vi "pdv_usb1.vi"() -> ()   [LabVIEW 2010]
uses:
  70user.lib/TheSigTab.vi
  <vilib>/Utility/config.llb/Read Key (U32).vi
  <vilib>/Utility/config.llb/Read Key (Boolean).vi
  <vilib>/Utility/config.llb/Read Key (Double).vi
  <vilib>/addons/database/Connection.llb/DB Tools Open Connec (Path).vi
  <vilib>/Utility/config.llb/Read Key (String).vi
  <vilib>/Utility/config.llb/Write Key (Double).vi
  <vilib>/Utility/config.llb/Write Key (U32).vi
  <vilib>/Utility/config.llb/Write Key (Boolean).vi
  <vilib>/addons/database/NI_Database_API.lvlib
  <vilib>/Utility/config.llb/NI_LVConfig.lvlib
panel:
  in  "ScopeToo":bool caption="Сохранять осциллограммы"
  in  "m_s":u16(ring) items=["мин", "сек"]
  in  "Object":string(combo) caption="Объект"
  in  "CurvesToo":bool caption="Сохранять графики"
  in  "AcqureTime":dbl caption="опроса" format="%#.3g"
  out "ExtDev":bool caption="Выносной модуль"
  in  "SaveTime":dbl=1.0 caption="мин" min=1.0 max=120.0
  out "Slide":u8(slide) scale=0.0..100.0
  in  "Continuosly":bool caption="Периодически"
  in  "SaveNow":bool caption="Однократно"
  in  "Loop":bool caption="Зациклить данные"
  out "Current time":timestamp caption="Время и Дата" format="%<%X\n%x>T"
  out "Tper":dbl caption="общая"
  in  "filter":bool caption="Фильтр\nперекрёстных помех"
  in  "Stop":bool
  in  "Table":string[][](table) caption="Результаты измерений"
  # "Запись в базу данных"
  # "Продолжительность, с"
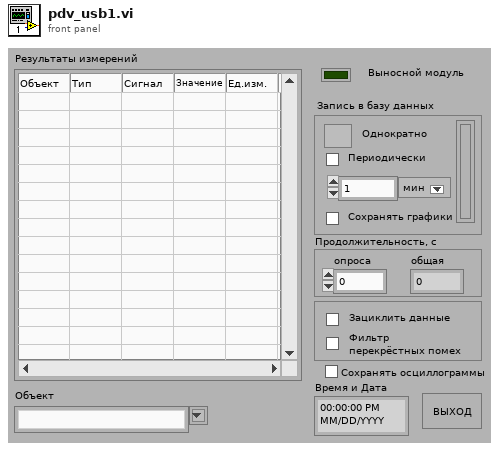
[diagram p1: front panel]
types:
  T1 = typedef "NI_LVConfig.lvlib/Config Data RefNum.ctl" = refnum<k1>
  T2 = typedef "NI_Database_API.lvlib/Conn ObjectReference.ctl" = refnum<k1>
  T3 = cluster{"Status":bool, "ViErrorNumber":u32, "ViName":string, "ViErrorString":string, "CinName":string, "CinErrorString":string}
  T4 = cluster{"VirtualSlot":u16, "ModuleName":string, "SerialNumber":string, "UsbSpeed":u8, "AvrVersion":string, "ModuleRevision":string, "DspType":string, "IsDacPresented":bool, "DspLoading":bool, "DspVersion":string, "DspClockout":u32, "AdcOffsetCoef":sgl[], "AdcScaleCoef":sgl[], "DacOffsetCoef":sgl[], "DacScaleCoef":sgl[]}
  T5 = cluster{"DllVersion":u32, "InterfaceType":u32, "InterfaceInstance":u32, "ModuleHandle":u32, "ReadBuffersParsArray":cluster{"Buffer":i16[], "ReadOv":u32, "ReadEvent":u32}[], "WriteBuffersParsArray":cluster{"Buffer":i16[], "WriteOv":u32, "WriteEvent":u32}[]}
  T6 = cluster{"Сигнал":string, "Тип":enum16{"Напряжение/Ток", "ЧР", "Температура", "Давление"}, "Object":string}[]
  T7 = cluster{"Сигнал":string, "Тип":enum16{"Напряжение/Ток", "ЧР", "Температура", "Давление"}, "Object":string}
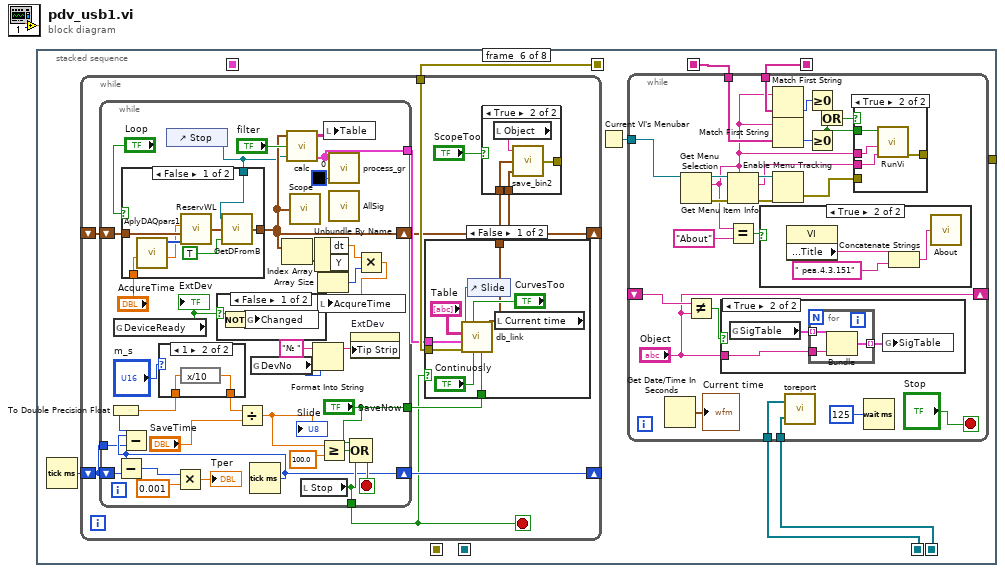
[diagram p0: block diagram]
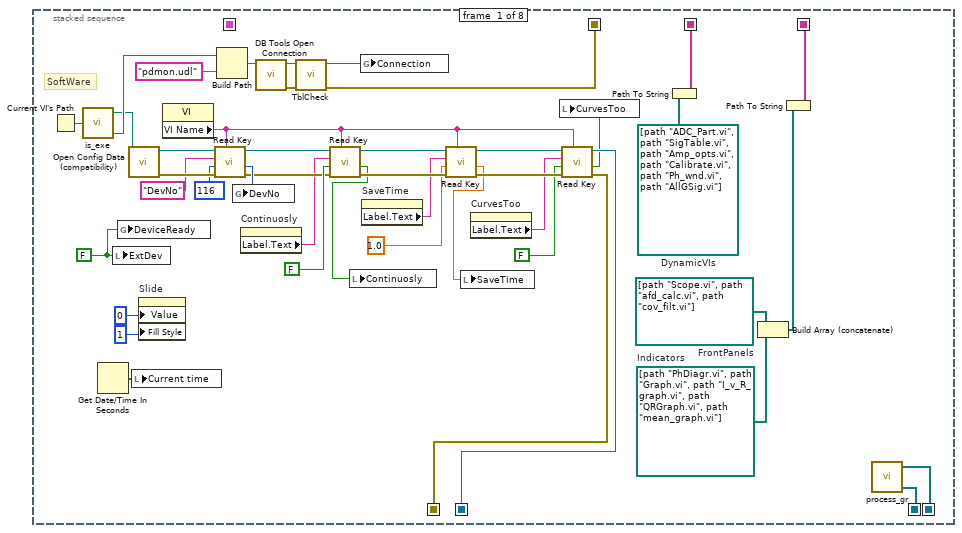
[diagram p2: hidden frame]
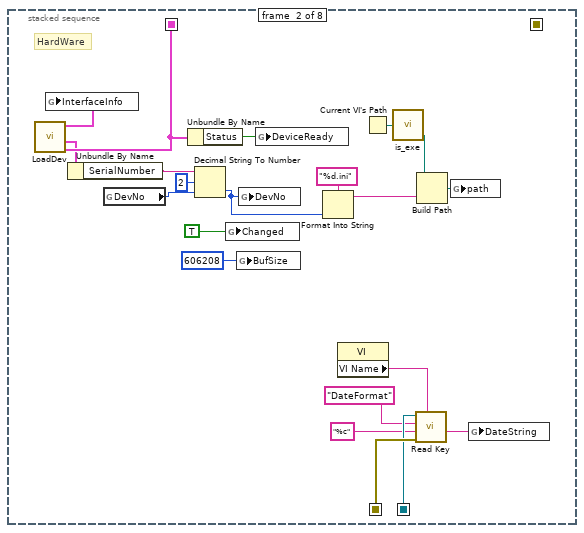
[diagram p3: hidden frame]
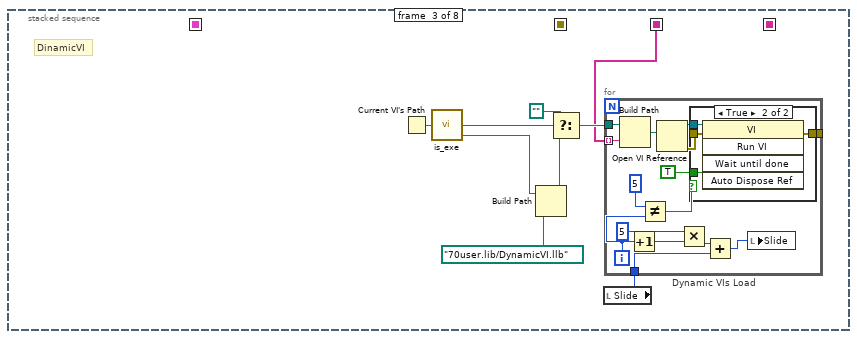
[diagram p4: hidden frame]
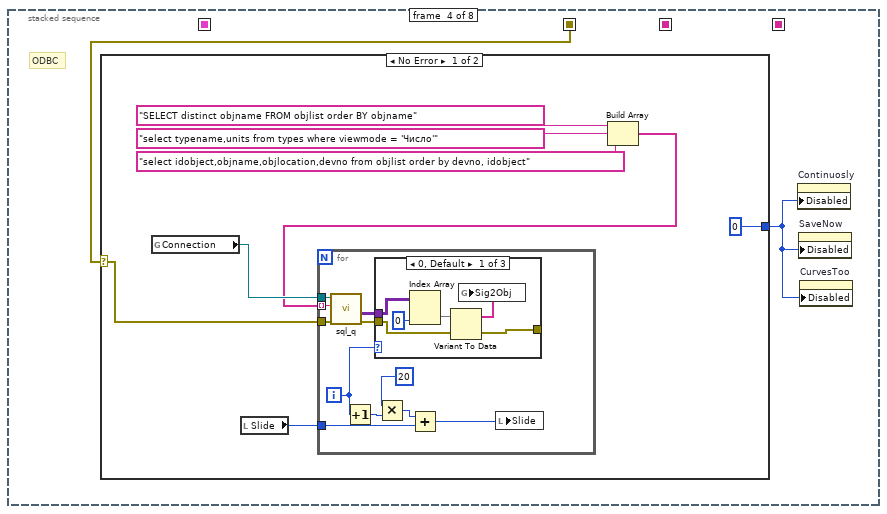
[diagram p6: hidden frame]
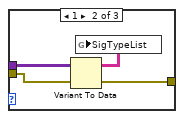
[diagram p7: hidden frame]
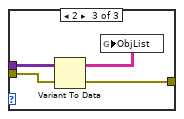
[diagram p8: hidden frame]
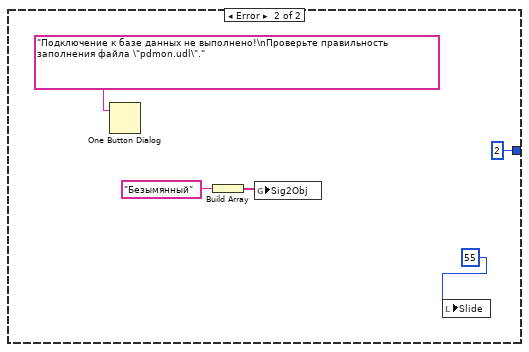
[diagram p9: hidden frame]
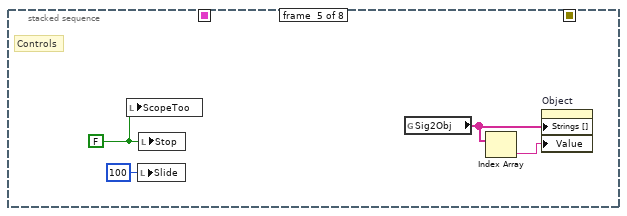
[diagram p10: hidden frame]
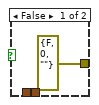
[diagram p11: hidden frame]
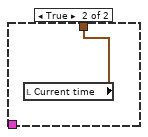
[diagram p12: hidden frame]
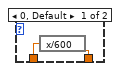
[diagram p13: hidden frame]
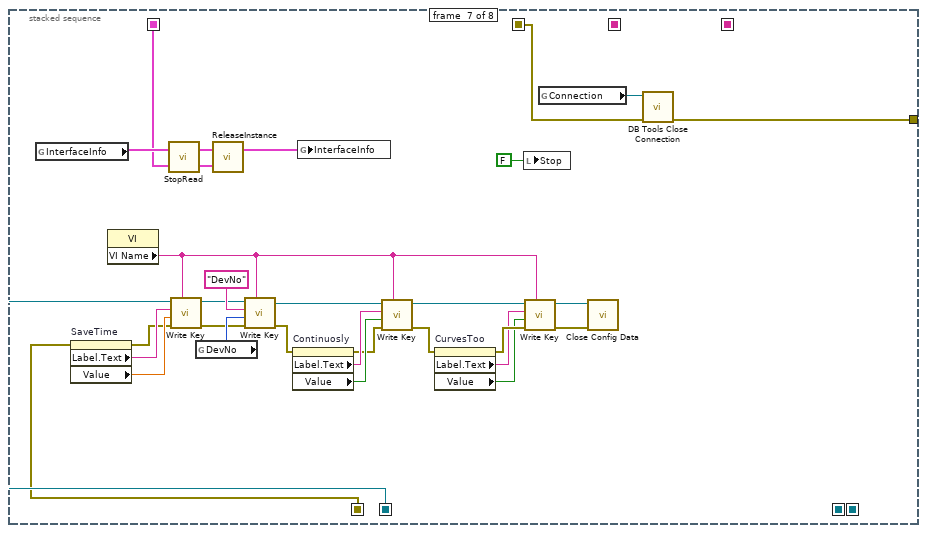
[diagram p19: hidden frame]
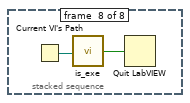
[diagram p20: hidden frame]
diagram:
  n1 = stacked-sequence {
    seq-local: [_ w60 _ _ _ _ _ _] -> [_ _ _ _ _ _ w282 _]
    seq-local: [w30 _ _ _ _ _ _ _] -> [_ _ _ w96 _ w144 w289 _]
    seq-local: [w33 _ _ _ _ _ _ _] -> [_ _ _ _ _ w142 _ _]
    seq-local: [w37 _ _ _ _ _ _ _] -> [_ _ w69 _ _ w141 _ _]
    seq-local: [w40 _ _ _ _ _ _ _] -> [_ _ _ _ _ w139 _ _]
    seq-local: [w39 _ _ _ _ _ _ _] -> [_ _ _ _ _ w140 _ _]
    seq-local: [w9 _ _ _ _ _ _ _] -> [_ w49 _ _ _ _ w274 _]
    seq-local: [w10 _ _ _ _ _ _ _] -> [_ w50 _ _ _ _ w268 _]
    tunnel: [_ _ _ _ _ _ w286 _] -> _
    frame #0 {
      w19 = FALSE ("ExtDev")
      w35 = path[] [path "PhDiagr.vi", path "Graph.vi", path "I_v_R_graph.vi", path "QRGraph.vi", path "mean_graph.vi"]  # Indicators
      w36 = path[] [path "Scope.vi", path "afd_calc.vi", path "cov_filt.vi"]  # FrontPanels
      w38 = path[] [path "ADC_Part.vi", path "SigTable.vi", path "Amp_opts.vi", path "Calibrate.vi", path "Ph_wnd.vi", path "AllGSig.vi"]  # DynamicVIs
      # "SoftWare"
      n2 = Current VI's Path() -> (path=w44:path)
      n3 = call "is_exe.vi"("path"=w44) -> ("actual path"=w43:path, "ini path"=w25:path)  [unwired: 2 in, 1 out]
      n4 = Get Date/Time In Seconds() -> (seconds since 1Jan1904=w28:timestamp)
      n5 = local write "ExtDev"(w19) -> ()
      n6 = global write "TheSigTab.vi" "DeviceReady"(w19) -> ()
      n7 = call <vilib>:"Open Config Data (compatibility).vi"("configuration file path"=w25) -> ("error out"=w23:errorcluster, "refnum"=w24:T1)  [unwired: 8 in, 1 out]
      n8 = local write "Current time"(w28) -> ()
      n9 = property on="Slide" class="Slide (strict)"("Value"=u8 0 ("Slide"), "Fill Style"=1) -> ()  [unwired: 2 in, 2 out]
      n10 = property class="VI"() -> ("VI Name"=w17:string)  [unwired: 2 in, 2 out]
      n11 = call-poly <vilib>:"Read Key.vi"("section"=w17, "error in (no error)"=w23, "default value"=u32 116 ("DevNo"), "key"="DevNo", "refnum"=w24) -> ("error out"=w15:errorcluster, "value"=w20:u32, "refnum out"=w18:T1)  [unwired: 3 in, 1 out]
      n12 = Build Path(base path=w43, name or relative path="pdmon.udl") -> (appended path=w41:path)
      n13 = global write "TheSigTab.vi" "DevNo"(w20) -> ()
      n14 = property on="Continuosly" class="Bool (strict)"() -> ("Label.Text"=w4:string)  [unwired: 2 in, 2 out]
      n15 = call-poly <vilib>:"DB Tools Open Connection.vi"("connection information"=w41) -> ("error out"=w31:errorcluster, "connection reference"=w32:T2)  [unwired: 7 in]
      n16 = call "TblCheck.vi"("error in"=w31, "connection reference"=w32) -> ("error out"=w30:errorcluster, "conn ref out"=w29:T2)  [unwired: 3 in, 1 out]
      n17 = call-poly <vilib>:"Read Key.vi"("section"=w17, "error in (no error)"=w15, "default value"=FALSE, "key"=w4, "refnum"=w18) -> ("error out"=w14:errorcluster, "value"=w2:bool, "refnum out"=w12:T1)  [unwired: 3 in, 1 out]
      n18 = local write "Continuosly"(w2) -> ()
      n19 = global write "TheSigTab.vi" "Connection"(w29) -> ()
      n20 = property on="SaveTime" class="DigNum (strict)"() -> ("Label.Text"=w3:string)  [unwired: 2 in, 2 out]
      n21 = call-poly <vilib>:"Read Key.vi"("section"=w17, "error in (no error)"=w14, "default value"=1.0, "key"=w3, "refnum"=w12) -> ("error out"=w13:errorcluster, "value"=w6:dbl, "refnum out"=w11:T1)  [unwired: 3 in, 1 out]
      n22 = local write "SaveTime"(w6) -> ()
      n23 = property on="CurvesToo" class="Bool (strict)"() -> ("Label.Text"=w1:string)  [unwired: 2 in, 2 out]
      n24 = call-poly <vilib>:"Read Key.vi"("section"=w17, "error in (no error)"=w13, "default value"=FALSE, "key"=w1, "refnum"=w11) -> ("error out"=w10:errorcluster, "value"=w5:bool, "refnum out"=w9:T1)  [unwired: 3 in, 1 out]
      n25 = local write "CurvesToo"(w5) -> ()
      n26 = Path To String(path=w38) -> (string=w37:string[])
      n27 = Build Array (concatenate)(w36, w35) -> (w34:path[])
      n28 = Path To String(path=w34) -> (string=w33:string[])
      n29 = call "process_gr.vi"() -> ("WG refs"=w40:refnum<vi>[], "menu refs"=w39:refnum<k9>[])  [unwired: 4 in]
    }
    frame #1 {
      # "HardWare"
      n30 = call "LoadDev.vi"() -> ("ViStatus"=w60:T3, "ModuleInfo"=w59:T4, "InterfaceInfo"=w61:T5)  [unwired: 5 in]
      n31 = global write "TheSigTab.vi" "InterfaceInfo"(w61) -> ()
      n32 = Unbundle By Name(w59) -> ("SerialNumber"=w58:string)
      n33 = global read "TheSigTab.vi" "DevNo"() -> (w51:u32)
      n34 = Unbundle By Name(w60) -> ("Status"=w65:bool)
      n35 = Decimal String To Number(string=w58, offset=u32 2 ("initial scan location"), default (0L)=w51) -> (number=w53:u32)  [unwired: 1 out]
      n36 = global write "TheSigTab.vi" "Changed"(TRUE ("Changed")) -> ()
      n37 = global write "TheSigTab.vi" "BufSize"(u32 606208 ("BufSize")) -> ()
      n38 = global write "TheSigTab.vi" "DevNo"(w53) -> ()
      n39 = global write "TheSigTab.vi" "DeviceReady"(w65) -> ()
      n40 = Format Into String(format string="%d.ini", w53) -> (resulting string=w55:string)  [unwired: 2 in, 1 out]
      n41 = property class="VI"() -> ("VI Name"=w48:string)  [unwired: 2 in, 2 out]
      n42 = Current VI's Path() -> (path=w64:path)
      n43 = call "is_exe.vi"("path"=w64) -> ("actual path"=w52:path)  [unwired: 2 in, 2 out]
      n44 = call-poly <vilib>:"Read Key.vi"("section"=w48, "error in (no error)"=w50, "default value"="%c", "key"="DateFormat", "refnum"=w49) -> ("value"=w45:string)  [unwired: 3 in, 3 out]
      n45 = Build Path(base path=w52, name or relative path=w55) -> (appended path=w54:path)
      n46 = global write "TheSigTab.vi" "path"(w54) -> ()
      n47 = global write "TheSigTab.vi" "DateString"(w45) -> ()
    }
    frame #2 {
      # "DinamicVI"
      n48 = Current VI's Path() -> (path=w68:path)
      n49 = call "is_exe.vi"("path"=w68) -> ("actual path"=w66:path, "exe?"=w67:bool)  [unwired: 2 in, 1 out]
      n50 = Build Path(base path=w66, name or relative path=path "70user.lib/DynamicVI.llb" ("f")) -> (appended path=w70:path)
      n51 = Select(t=path "", s=w67, f=w70) -> (s? t:f=w74:path)
      n52 = local read "Slide"() -> (w73:u8)
      n53 = for "Dynamic VIs Load" {
        tunnel: w69 -> [w89] mode=indexing
        tunnel: w74 -> [w87]
        tunnel: w73 -> [w83]
        tunnel: [w78] -> _
        i -> [w77]
        n54 = Build Path(base path=w87, name or relative path=w89) -> (appended path=w88:path)
        n55 = Increment(x=w77) -> (x+1=w79:i32)
        n56 = Not Equal?(x=5, y=w77) -> (x != y?=w75:bool)
        n57 = Open VI Reference(vi path=w88) -> (vi reference=w85:refnum<vi>, error out=w84:errorcluster)  [unwired: 5 in]
        n58 = Multiply(x=5, y=w79) -> (x*y=w81:i32)
        n59 = case shown="True" w75 {
          tunnel: TRUE ("Wait until done") -> [_ w94]
          tunnel: w85 -> [_ w93]
          tunnel: w84 -> [w90 w92]
          tunnel: [w90 w91] -> w78
          frame False {
          }
          frame True {
            n60 = invoke class="VI" method="Run VI"(reference=w93, error in=w92, "Wait until done"=w94) -> (error out=w91:errorcluster)  [unwired: 2 in, 4 out]
          }
        }
        n61 = Add(x=w81, y=w83) -> (x+y=w82:i32)
        n62 = local write "Slide"(w82) -> ()
      }
    }
    frame #3 {
      # "ODBC"
      n63 = case shown="No Error" w96 {
        selector: w96 -> [w100 _]
        tunnel: [u8 0 ("Disabled") u8 2 ("Disabled")] -> w95
        frame No Error {
          n64 = global read "TheSigTab.vi" "Connection"() -> (w101:T2)
          n65 = local read "Slide"() -> (w98:u8)
          n66 = Build Array("SELECT distinct objname FROM objlist order BY objname", "select typename,units from types where viewmode = 'Число'", "select idobject,objname,objlocation,devno from objlist order by devno, idobject" ("table")) -> (w99:string[])
          n67 = for {
            tunnel: w101 -> [w114]
            tunnel: w100 -> [w113]
            tunnel: w99 -> [w111] mode=indexing
            tunnel: w98 -> [w110]
            i -> [w107]
            n68 = call "sql_q.vi"("error in"=w113, "SQL query"=w111, "connect ref"=w114) -> ("error out"=w112:errorcluster, "recordset data"=w115:variant[][])  [unwired: 1 in, 2 out]
            n69 = Increment(x=w107) -> (x+1=w105:i32)
            n70 = case shown="0, Default" w107 {
              tunnel: w115 -> [w118 w125 w129]
              tunnel: w112 -> [w117 w123 w127]
              tunnel: [w116 w122 w126] -> _
              frame 0, Default {
                n71 = Index Array(array=w118, index (col)=0 ("disabled index (col)")) -> (element=w120:variant[])  [unwired: 1 in]
                n72 = Variant To Data(error in=w117, Variant=w120) -> (error out=w116:errorcluster, data=w119:string[])  [unwired: 1 in]
                n73 = global write "TheSigTab.vi" "Sig2Obj"(w119) -> ()
              }
              frame 1 {
                n74 = Variant To Data(error in=w123, Variant=w125) -> (error out=w122:errorcluster, data=w124:string[][])  [unwired: 1 in]
                n75 = global write "TheSigTab.vi" "SigTypeList"(w124) -> ()
              }
              frame 2 {
                n76 = Variant To Data(error in=w127, Variant=w129) -> (error out=w126:errorcluster, data=w128:string[][])  [unwired: 1 in]
                n77 = global write "TheSigTab.vi" "ObjList"(w128) -> ()
              }
            }
            n78 = Multiply(x=20, y=w105) -> (x*y=w108:i32)
            n79 = Add(x=w108, y=w110) -> (x+y=w109:i32)
            n80 = local write "Slide"(w109) -> ()
          }
        }
        frame Error {
          n81 = One Button Dialog(message="Подключение к базе данных не выполнено!\nПроверьте правильность заполнения файла \"pdmon.udl\".") -> ()  [unwired: 1 in, 1 out]
          n82 = Build Array("Безымянный" ("table")) -> (w133:string[])
          n83 = global write "TheSigTab.vi" "Sig2Obj"(w133) -> ()
          n84 = local write "Slide"(u8 55 ("Slide")) -> ()
        }
      }
      n85 = property on="Continuosly" class="Bool (strict)"("Disabled"=w95) -> ()  [unwired: 2 in, 2 out]
      n86 = property on="SaveNow" class="Bool"("Disabled"=w95) -> ()  [unwired: 2 in, 2 out]
      n87 = property on="CurvesToo" class="Bool (strict)"("Disabled"=w95) -> ()  [unwired: 2 in, 2 out]
    }
    frame #4 {
      w135 = FALSE ("Changed")
      # "Controls"
      n88 = local write "ScopeToo"(w135) -> ()
      n89 = local write "Slide"(u8 100 ("Slide")) -> ()
      n90 = local write "Stop"(w135) -> ()
      n91 = global read "TheSigTab.vi" "Sig2Obj"() -> (w137:string[])
      n92 = Index Array(array=w137) -> (element=w136:string)  [unwired: 1 in]
      n93 = property on="Object" class="CmbBox"("Strings []"=w137, "Value"=w136) -> ()  [unwired: 2 in, 2 out]
    }
    frame #5 {
      n94 = Tick Count (ms)() -> (millisecond timer value=w145:u32)
      n95 = while {
        shift-right: [w155] -> _
        shift-left: w145 -> [w152]
        shift-right: [w148] -> _
        shift-left: _ -> [w154]
        tunnel: w144 -> [w153]
        stop <- w149 stop-if-true
        n96 = while {
          shift-right: [w182] -> w148
          shift-left: w154 -> [w201]
          shift-right: [w196] -> w155
          shift-left: w152 -> [w202]
          tunnel: [w198] -> w149
          tunnel: w152 -> [w195]
          tunnel: ["SaveNow"] -> w151
          tunnel: [w188] -> w150
          stop <- w197 stop-if-true
          n97 = global read "TheSigTab.vi" "DeviceReady"() -> (w193:bool)
          "ExtDev" <- w193
          n98 = control-ref of="Stop"() -> (w176:refnum<vi>)
          n99 = case shown="False" "Loop" {
            tunnel: w201 -> [w218 w219]
            tunnel: [w215 w219] -> w182
            tunnel: "AcqureTime" -> [w212 _]
            tunnel: w176 -> [w211 _]
            frame False {
              n100 = call "AplyDAQpars1.vi"("AcqTimeIn"=w212) -> ("t1-t0"=w213:dbl, "Idxs"=w217:i32[])  [unwired: 5 in]
              n101 = call "ReservWL.vi"("Tags"=w217, "ArrayIn"=w218, "t1-t0"=w213) -> ("Array"=w216:waveform(i16)[])  [unwired: 1 in]
              n102 = call "GetDFromB.vi"("Control"=TRUE, "ArrayIn"=w216, "Bool Refnum"=w211) -> ("ArrayOut"=w215:waveform(i16)[])
            }
            frame True {
            }
          }
          n103 = case shown="False" w193 {
            selector: w193 -> [w210 _]
            frame False {
              n104 = Not(x=w210) -> (.not. x?=w209:bool)
              n105 = global write "TheSigTab.vi" "Changed"(w209) -> ()
            }
            frame True {
            }
          }
          n106 = Tick Count (ms)() -> (millisecond timer value=w196:u32)
          n107 = Subtract(x=w196, y=w202) -> (x-y=w192:u32)
          n108 = Subtract(x=w196, y=w195) -> (x-y=w194:u32)
          n109 = To Double Precision Float(number=w194) -> (double precision float=w171:dbl)
          n110 = case shown="1" "m_s" {
            tunnel: w171 -> [w206 w208]
            tunnel: [w205 w207] -> w170
            frame 0, Default {
              n111 = expression code="x/600"(w206) -> (w205:dbl)
            }
            frame 1 {
              n112 = expression code="x/10"(w208) -> (w207:dbl)
            }
          }
          n113 = Multiply(x=w192, y=0.001 ("x")) -> (x*y=→"Tper":dbl)
          n114 = Divide(x=w170, y="SaveTime") -> (x/y=w186:dbl)
          "Slide" <- w186
          n115 = global read "TheSigTab.vi" "DevNo"() -> (w173:u32)
          n116 = Index Array(array=w182) -> (element=w181:waveform(i16))  [unwired: 1 in]
          n117 = call "calc.vi"("Acquire"=w176, "filter"="filter", "ArrayIn"=w182) -> ("AllMeasures"=w188:cluster{"x0":dbl, "dx":dbl, "y":sgl[][]}[], "Values"=w204:string[][])  [unwired: 1 in]
          n118 = call "Scope.vi"("Array"=w182) -> ()
          n119 = local read "Stop"() -> (w198:bool)
          n120 = Format Into String(initial string="№ ", w173) -> (resulting string=w175:string)  [unwired: 2 in, 1 out]
          n121 = Unbundle By Name(w181) -> ("dt"=w179:dbl, "Y"=w180:i16[])
          n122 = Array Size(array=w180) -> (size(s)=w178:i32)
          n123 = Greater Or Equal?(x=w186, y=100.0 ("x")) -> (x >= y?=w183:bool)
          n124 = local write "Table"(w204) -> ()
          n125 = call "process_gr.vi"("Color Box"=u32 0, "AllMeasures"=w188) -> ()  [unwired: 2 in, 2 out]
          n126 = call "AllSig.vi"() -> ()  [unwired: 1 in]
          n127 = Compound Arithmetic op=OR("SaveNow", w183, w198) -> (w197:bool)
          n128 = property on="ExtDev" class="Bool (strict)"("Tip Strip"=w175) -> ()  [unwired: 2 in, 2 out]
          n129 = Multiply(x=w179, y=w178) -> (x*y=w177:dbl)
          n130 = local write "AcqureTime"(w177) -> ()
        }
        n131 = case shown="False" w149 {
          tunnel: w153 -> [w168 _]
          tunnel: w151 -> [w167 _]
          tunnel: w150 -> [w165 _]
          tunnel: [w161 w169] -> w147
          frame False {
            n132 = control-ref of="Slide"() -> (w164:refnum<vi>)
            n133 = local read "Current time"() -> (w161:timestamp)
            n134 = call "db_link.vi"("Current time"=w161, "SaveNow"=w167, "Continuosly"="Continuosly", "SaveCurves?"="CurvesToo", "error in"=w168, "AllMeasures"=w165, "Table"="Table", "reference"=w164) -> ()  [unwired: 3 in, 1 out]
          }
          frame True {
            n135 = local read "Current time"() -> (w169:timestamp)
          }
        }
        n136 = case shown="True" "ScopeToo" {
          tunnel: [errorcluster {"status"=FALSE, "code"=0, "source"=""} ("error out") w160] -> _
          tunnel: w148 -> [_ w159]
          tunnel: w147 -> [_ w158]
          frame False {
          }
          frame True {
            n137 = local read "Object"() -> (w157:string)
            n138 = call "save_bin2.vi"("ArrayOut"=w159, "Current time"=w158, "Object"=w157) -> ("error out"=w160:errorcluster)
          }
        }
      }
      n139 = Current VI's Menubar() -> (w143:refnum<k9>)
      n140 = while {
        tunnel: w143 -> [w241]
        tunnel: w142 -> [w237]
        tunnel: w141 -> [w234]
        tunnel: w140 -> [w232]
        tunnel: w139 -> [w231]
        shift-right: ["Object"] -> _
        shift-left: _ -> [w224]
        stop <- "Stop" stop-if-true
        n141 = Get Date/Time In Seconds() -> (seconds since 1Jan1904=→"Current time":timestamp)
        n142 = Get Menu Selection(0:w241) -> (5:w240:refnum<k9>, 6:w222:string, 8:w233:errorcluster)  [unwired: 3 in, 2 out]
        n143 = Not Equal?(x=w224, y="Object") -> (x != y?=w225:bool)
        n144 = case shown="True" w225 {
          tunnel: "Object" -> [_ w248]
          frame False {
          }
          frame True {
            n145 = global read "TheSigTab.vi" "SigTable"() -> (w250:T6)
            n146 = for {
              tunnel: w250 -> [w253] mode=indexing
              tunnel: w248 -> [w252]
              tunnel: [w251] -> w249 mode=indexing
              n147 = Bundle(cluster=w253, "Object"=w252) -> (w251:T7)  [unwired: 2 in]
            }
            n148 = global write "TheSigTab.vi" "SigTable"(w249) -> ()
          }
        }
        n149 = Get Menu Item Info(7:w222, 8:w233, 11:w240) -> (0:w230:errorcluster, 2:w236:string, 3:w239:refnum<k9>)  [unwired: 4 out]
        n150 = Equal?(x=w222, y="About") -> (x = y?=w220:bool)
        n151 = case shown="True" w220 {
          frame False {
          }
          frame True {
            n152 = property class="VI"() -> ("Front Panel Window:Title"=w247:string)  [unwired: 2 in, 2 out]
            n153 = Concatenate Strings(w247, " рев.4.3.151" ("input 1")) -> (w245:string)
            n154 = call "About.vi"("Revision Number"=w245) -> ()
          }
        }
        n155 = Match First String(2:w237, 3:w222) -> (0:w238:i32)  [unwired: 1 out]
        n156 = Match First String(2:w234, 3:w222) -> (0:w235:i32)  [unwired: 1 out]
        n157 = Enable Menu Tracking(2:w230, 4:w239) -> (0:w226:errorcluster)  [unwired: 1 in, 1 out]
        n158 = call "toreport.vi"("Menu"=w232, "WG"=w231) -> ()
        n159 = Greater Or Equal To 0?(x=w238) -> (x >= 0?=w229:bool)
        n160 = Greater Or Equal To 0?(x=w235) -> (x >= 0?=w228:bool)
        n161 = Or(x=w229, y=w228) -> (x .or. y?=w227:bool)
        n162 = case shown="True" w227 {
          tunnel: w236 -> [_ w258]
          tunnel: w222 -> [_ w257]
          tunnel: w228 -> [_ w256]
          tunnel: w226 -> [w254 _]
          tunnel: [w254 w255] -> _
          frame False {
          }
          frame True {
            n163 = call "RunVi.vi"("Title"=w258, "Name"=w257, "Run/JustOpen"=w256) -> ("error out"=w255:errorcluster)  [unwired: 4 in]
          }
        }
        n164 = Wait (ms)(milliseconds to wait=u32 125) -> ()  [unwired: 1 out]
      }
    }
    frame #6 {
      n165 = global read "TheSigTab.vi" "InterfaceInfo"() -> (w284:T5)
      n166 = property on="SaveTime" class="DigNum (strict)"(error in=w268) -> (error out=w269:errorcluster, "Label.Text"=w276:string, "Value"=w275:dbl)  [unwired: 1 in, 1 out]
      n167 = property class="VI"() -> ("VI Name"=w259:string)  [unwired: 2 in, 2 out]
      n168 = call "StopRead.vi"("ViStatusIn"=w282, "InterfaceInfoIn"=w284) -> ("ViStatusOut"=w281:T3, "InterfaceInfoOut"=w283:T5)
      n169 = call-poly <vilib>:"Write Key.vi"("section"=w259, "error in (no error)"=w269, "value"=w275, "key"=w276, "refnum"=w274) -> ("error out"=w277:errorcluster, "refnum out"=w278:T1)  [unwired: 4 in, 1 out]
      n170 = global read "TheSigTab.vi" "DevNo"() -> (w280:u32)
      n171 = call "ReleaseInstance.vi"("ViStatusIn"=w281, "InterfaceInfoIn"=w283) -> ("InterfaceInfoOut"=w285:T5)  [unwired: 1 out]
      n172 = call-poly <vilib>:"Write Key.vi"("section"=w259, "error in (no error)"=w277, "value"=w280, "key"="DevNo", "refnum"=w278) -> ("error out"=w267:errorcluster, "refnum out"=w273:T1)  [unwired: 4 in, 1 out]
      n173 = property on="Continuosly" class="Bool (strict)"(error in=w267) -> (error out=w266:errorcluster, "Label.Text"=w272:string, "Value"=w271:bool)  [unwired: 1 in, 1 out]
      n174 = global write "TheSigTab.vi" "InterfaceInfo"(w285) -> ()
      n175 = call-poly <vilib>:"Write Key.vi"("section"=w259, "error in (no error)"=w266, "value"=w271, "key"=w272, "refnum"=w273) -> ("error out"=w265:errorcluster, "refnum out"=w264:T1)  [unwired: 4 in, 1 out]
      n176 = property on="CurvesToo" class="Bool (strict)"(error in=w265) -> (error out=w270:errorcluster, "Label.Text"=w263:string, "Value"=w262:bool)  [unwired: 1 in, 1 out]
      n177 = local write "Stop"(FALSE ("Stop")) -> ()
      n178 = call-poly <vilib>:"Write Key.vi"("section"=w259, "error in (no error)"=w270, "value"=w262, "key"=w263, "refnum"=w264) -> ("error out"=w261:errorcluster, "refnum out"=w260:T1)  [unwired: 4 in, 1 out]
      n179 = global read "TheSigTab.vi" "Connection"() -> (w288:T2)
      n180 = call <vilib>:"Close Config Data.vi"("error in (no error)"=w261, "refnum"=w260) -> ()  [unwired: 8 in, 2 out]
      n181 = call <vilib>:"DB Tools Close Connection.vi"("error in (no error)"=w289, "connection reference"=w288) -> ("error out"=w286:errorcluster)  [unwired: 5 in]
    }
    frame #7 {
      n182 = Current VI's Path() -> (path=w290:path)
      n183 = call "is_exe.vi"("path"=w290) -> ("exe?"=w291:bool)  [unwired: 2 in, 2 out]
      n184 = Quit LabVIEW(quit? (T)=w291) -> ()
    }
  }
